vi "Actor Core.vi"(8 "error in":errorcluster, 11 "DATABASE in":refnum<class "DATABASE.lvclass">) -> (0 "error out":errorcluster, 3 "Actor out":refnum<class "Actor.lvclass">)   [LabVIEW 2019, in "DATABASE.lvlib" / "DATABASE.lvclass"]
doc: "(<B>Filename</B>: Actor Framework.lvlib:Actor.lvclass:Actor Core.vi)\n\nReceives messages to the actor, reacts to them, and initiates any error handling that may shut the actor down.\n\nDescendant classes may override this VI to append parallel tasks for the actor to complete while it handles messages. Overrides use the Call Parent Method node."
uses:
  DATABASE.lvclass
  C:/Program Files (x86)/National Instruments/LabVIEW 2019/vi.lib/ActorFramework/Actor/Actor.lvclass
  <vilib>/ActorFramework/Actor/Actor.lvclass
  <vilib>/ActorFramework/Actor/Actor.lvclass/Actor.ctl
  DATABASE.lvclass/DATABASE.ctl
  CAFE_MEX_ESP Messages/SOLOCITAR MERCANCIA Msg/SOLOCITAR MERCANCIA Msg.lvclass/SOLOCITAR MERCANCIA Msg.ctl
  <vilib>/ActorFramework/Message Enqueuer/Message Enqueuer.lvclass/Message Enqueuer.ctl
  <vilib>/drjdpowell/SQLite Library/SQL Connection/Open (path).vi
  <vilib>/drjdpowell/SQLite Library/SQL Connection/Open (string).vi
  <vilib>/ActorFramework/Message Enqueuer/Enqueue.vi
  CAFE_MEX_ESP Messages/SOLOCITAR MERCANCIA Msg/SOLOCITAR MERCANCIA Msg.lvclass
  C:/Program Files (x86)/National Instruments/LabVIEW 2019/vi.lib/ActorFramework/Message/Message.lvclass
  <vilib>/AdvancedString/Path To Command Line String.vi
  <vilib>/drjdpowell/SQLite Library/SQL Connection/Execute SQL.vi
  <vilib>/ActorFramework/Message Priority Queue/Priority Enqueue.vi
  <vilib>/drjdpowell/SQLite Library/SQL Connection/Connection.lvclass
  <vilib>/drjdpowell/SQLite Library/SQLite.lvlib
panel:
  out "appended array":string[][](array[string])
  out "BASE_DE_DATOS":string
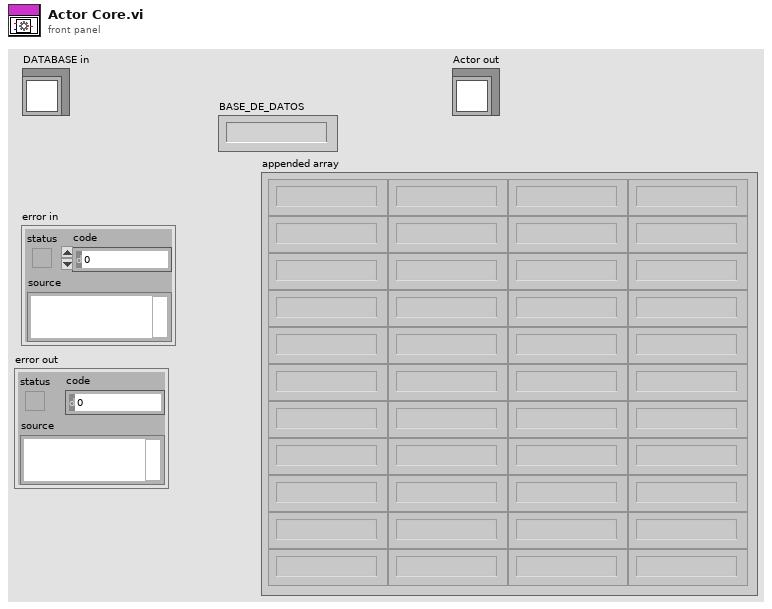
[diagram p1: front panel]
types:
  T1 = cluster{"BASE_DE_DATOS":refnum<user-event>, "EXIT":refnum<user-event>}
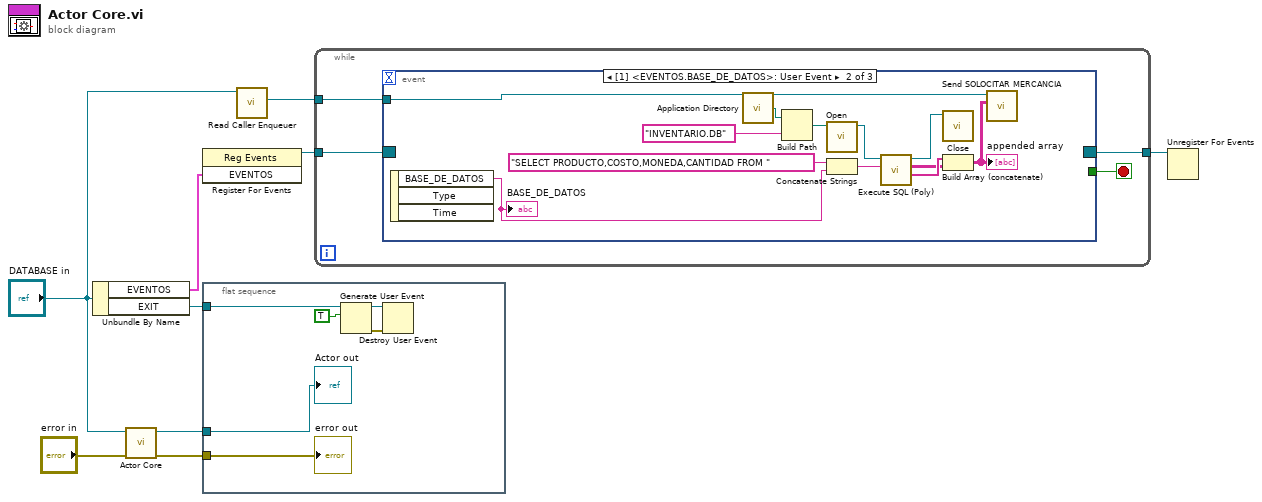
[diagram p0: block diagram]
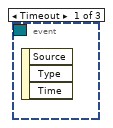
[diagram p2: hidden frame]
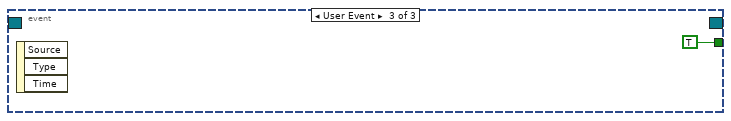
[diagram p3: hidden frame]
diagram:
  n1 = Unbundle By Name("DATABASE in") -> ("EVENTOS"=w8:T1, "EXIT"=w4:refnum<user-event>)
  n2 = call-parent "Actor Core.vi"("error in"="error in", "Actor in"="DATABASE in") -> ("error out"=w6:errorcluster, "Actor out"=w5:refnum<class "Actor.lvclass">)  [unwired: 8 in]
  n3 = register-events(w8) -> (reference out=w7:refnum<event-registration>)  [unwired: 2 in, 1 out]
  n4 = flat-sequence {
    tunnel: w6 -> [w15]
    tunnel: w5 -> [w14]
    tunnel: w4 -> [w11]
    frame #0 {
      n5 = Generate User Event(user event=w11, event data cluster=TRUE ("event data")) -> (user event out=w13:refnum<user-event>, error out=w12:errorcluster)  [unwired: 2 in]
      n6 = Destroy User Event(user event=w13, error in=w12) -> ()  [unwired: 1 out]
      "error out" <- w15
      "Actor out" <- w14
    }
  }
  n7 = call <vilib>:"Read Caller Enqueuer.vi"("Actor"="DATABASE in") -> ("Caller Enqueuer"=w1:refnum<class "Message Enqueuer.lvclass">)  [unwired: 10 in]
  n8 = while {
    tunnel: w7 -> [w19]
    tunnel: [w17] -> w3
    tunnel: w1 -> [w16]
    stop <- w18 stop-if-true
    n9 = event shown="[1] <EVENTOS.BASE_DE_DATOS>: User Event" {
      selector: w19 -> [_ _ _]
      dyn-events: [_ _ _] -> w17
      timeout: _ -> [_ _ _]
      tunnel: [_ _ TRUE] -> w18
      tunnel: w16 -> [_ w20 _]
      event Timeout {
        n10 = event-data() -> ()  [unwired: 1 in, 3 out]
      }
      event User Event {
        n11 = event-data() -> ("BASE_DE_DATOS"=w23:string)  [unwired: 1 in, 2 out]
        "BASE_DE_DATOS" <- w23
        n12 = call <vilib>:"Application Directory.vi"() -> ("Application Directory"=w31:path)
        n13 = Build Path(base path=w31, name or relative path="INVENTARIO.DB") -> (appended path=w30:path)
        n14 = call-poly <vilib>:"Open.vi"("db file"=w30) -> ("SQLite Connection"=w29:refnum<class "Connection.lvclass">)  [unwired: 9 in, 1 out]
        n15 = Concatenate Strings("SELECT PRODUCTO,COSTO,MONEDA,CANTIDAD FROM " ("string"), w23) -> (w22:string)
        n16 = call-poly <vilib>:"Execute SQL (Poly).vi"("SQL"=w22, "SQLite Connection in"=w29) -> ("Column Names"=w27:string[], "Result Set"=w26:string[][], "SQLite Connection"=w28:refnum<class "Connection.lvclass">)  [unwired: 6 in, 1 out]
        n17 = call-dynamic "Close.vi"("SQLite Connection in"=w28) -> ()  [unwired: 10 in, 1 out]
        n18 = Build Array (concatenate)(w27, w26) -> (w21:string[][])
        "appended array" <- w21
        n19 = call "Send SOLOCITAR MERCANCIA.vi"("appended array"=w21, "Message Enqueuer"=w20) -> ()  [unwired: 8 in, 2 out]
      }
      event User Event {
        n20 = event-data() -> ()  [unwired: 1 in, 3 out]
      }
    }
  }
  n21 = Unregister For Events(event registration refnum=w3) -> ()  [unwired: 1 in, 1 out]
